vi "Send Local Messages.vi"(0 "message queue in":T2, 1 "receiver process (\"\" - local)":string, 5 "message names":string[](array[string]), 7 "message values":string[](array[string]), 9 "timeout (-1 ms)":i32=-1, 11 "error in":errorcluster, 12 "message attributes":T1[](array[typedef])) -> (4 "message queue out":T2, 10 "timed out?":bool[](array[boolean]), 15 "error out":errorcluster)   [LabVIEW 2015, in "Car Wash.lvlib" / "AMC.lvlib"]
doc: "Adds one or more messages to the local message queue provided by the queue reference or to another message queue in the local application based on the receiver process name."
uses:
  AMC.lvlib
  Message Queue.ctl
  Message.ctl
  Tools/Keyed Array/KeyedArray.ctl
  Create Single Message.vi
  Tools/Keyed Array/Tools_KeyedArray.lvlib
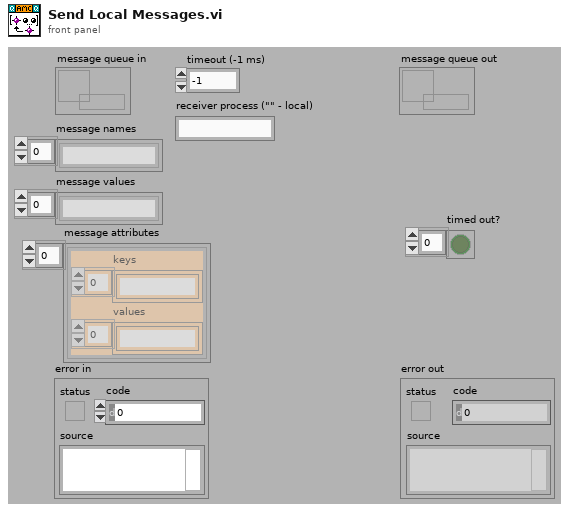
[diagram p1: front panel]
types:
  T1 = typedef "Car Wash.lvlib/Tools_KeyedArray.lvlib/KeyedArray.ctl" = cluster{"keys":string[], "values":string[]}
  T2 = typedef "Car Wash.lvlib/AMC.lvlib/Message Queue.ctl" = refnum<queue>
  T3 = typedef "Car Wash.lvlib/AMC.lvlib/Message.ctl" = cluster{"name":string, "value":string, "attributes":T1, "receiver host":string, "receiver process":string, "source host":string, "source process":string, "priority message":bool, "acknowledge message":bool}
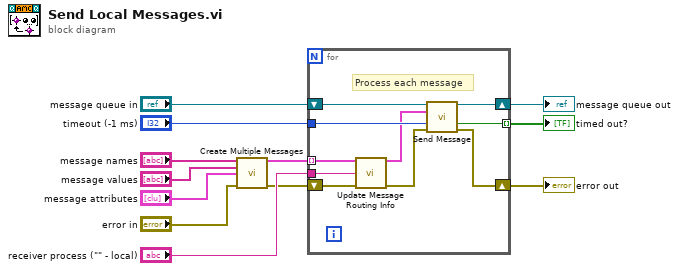
[diagram p0: block diagram]
diagram:
  n1 = call "Create Multiple Messages.vi"("names"="message names", "values"="message values", "attributes"="message attributes", "error in"="error in") -> ("messages"=w10:T3[], "error out"=w1:errorcluster)  [unwired: 10 in]
  n2 = for {
    shift-right: [w21] -> w11
    shift-left: "message queue in" -> [w22]
    tunnel: w10 -> [w17] mode=indexing
    shift-right: [w20] -> w6
    shift-left: w1 -> [w14]
    tunnel: "timeout (-1 ms)" -> [w19]
    tunnel: [w18] -> w4 mode=indexing
    tunnel: "receiver process (\"\" - local)" -> [w15]
    # "Process each message"
    n3 = call "Update Message Routing Info.vi"("message"=w17, "receiver process (\"\")"=w15, "error in"=w14) -> ("message"=w16:T3, "error out"=w13:errorcluster)  [unwired: 11 in]
    n4 = call "Send Message.vi"("message queue in"=w22, "message"=w16, "timeout (-1 ms)"=w19, "error in"=w13) -> ("message queue out"=w21:T2, "timed out?"=w18:bool, "error out"=w20:errorcluster)  [unwired: 9 in]
  }
  "message queue out" <- w11
  "error out" <- w6
  "timed out?" <- w4
